vi "ConfigureDlg.vi"(8 "error in (no error)":errorcluster, 11 "SiemensDigitalEnergyMeter in":refnum<class "SiemensDigitalEnergyMeter.lvclass">) -> (0 "error out":errorcluster, 2 "Changed":bool, 3 "SiemensDigitalEnergyMeter out":refnum<class "SiemensDigitalEnergyMeter.lvclass">)   [LabVIEW 2018, in "SensorPlugins.lvlib" / "SiemensDigitalEnergyMeter.lvclass"]
doc: "This VI allows the user to configure the instrument using the provided panel and saves the instruments configuration to file, a new file, or cancels the entire operation."
uses:
  SiemensDigitalEnergyMeter.lvclass
  C:/Program Files (x86)/National Instruments/LabVIEW 2018/user.lib/NIST/BaseClasses/BasePlugin_class/BasePlugin.lvclass
  TypeDefinitions/SiemensDigitalEnergyMeterControls.ctl
  TypeDefinitions/MeasurementControls.ctl
  <userlib>/NIST/BaseClasses/BasePlugin_class/BasePlugin.lvclass/BasePlugin.ctl
  <userlib>/NIST/BaseClasses/BasePlugin_class/Accessors/Read PluginIniFilePath.vi
  <userlib>/NIST/BaseClasses/BasePlugin_class/Accessors/Write PluginIniFilePath.vi
  <vilib>/Utility/config.llb/NI_LVConfig.lvlib
panel:
  in  "MeasurementCluster":T1
  in  "Siemens Digital Energy Meter":T2 {"Measurement(s)" items=["kWh System"=4000, "kVARh System"=4007, "kVAh System"=4010, "kVA System"=4012, "Volts L1 to L2"=4018, "Volts L2 to L3"=4019, "Volts L1 to L2"=4020, "Line Frequency"=4021, "kW L1"=4028, "kW L2"=4029, "kW L3"=4030, "kVAR L1"=4037, "kVAR L2"=4038, "kVAR L3"=4039, "kVA L1"=4046, "kVA L2"=4047, "kVA L3"=4048, "Apparent PF L1"=4052, "Apparent PF L2"=4053, "Apparent PF L3"=4054, "Amps L1"=4055, "Amps L2"=4056, "Amps L3"=4057, "Volts L1 to Neutral"=4058, "Volts L2 to Neutral"=4059, "Volts L3 to Neutral"=4060, "Firmware Major Revision"=4068, "Firmware Minor Revision "=4069, "Model Number "=4200, "Serial Number"=4205, "Hardware ID"=4510]}
  in  "btnSaveAs":bool
  in  "btnSave":bool
  in  "btnCancel":bool
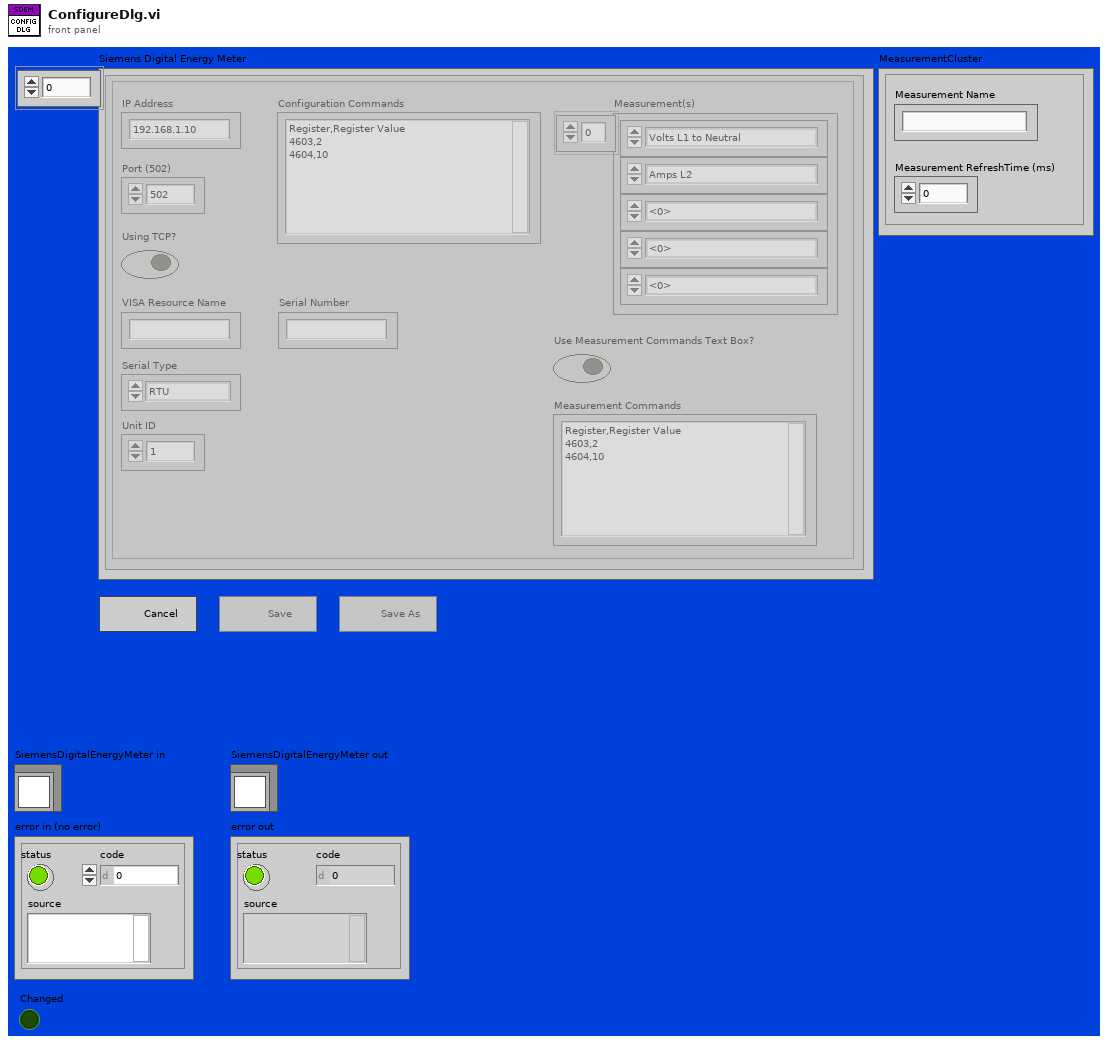
[diagram p1: front panel]
types:
  T1 = typedef "SensorPlugins.lvlib/SiemensDigitalEnergyMeter.lvclass/MeasurementControls.ctl" = cluster{"Measurement RefreshTime (ms)":u32, "Measurement Name":string}
  T2 = typedef "SensorPlugins.lvlib/SiemensDigitalEnergyMeter.lvclass/SiemensDigitalEnergyMeterControls.ctl" = cluster{"Measurement(s)":u16[], "Configuration Commands":string, "Use Measurement Commands Text Box?":bool, "Measurement Commands":string, "Connected?":bool, "Serial Number":string, "IP Address":string, "Port (502)":u16, "Unit ID":u8, "Serial Type":enum16{"RTU", "ASCII"}, "Using TCP?":bool, "VISA Resource Name":string}[]
  T3 = enum32{"Invalid", "Default", "Floating", "Floating/Auto-Hide", "Modal"}
  T4 = enum32{"Invalid", "Standard", "Closed", "Hidden", "Minimized", "Maximized"}
  T5 = enum8{"Enabled", "Disabled", "Disabled and Grayed Out"}
  T6 = cluster{"Measurement(s)":u16[], "Configuration Commands":string, "Use Measurement Commands Text Box?":bool, "Measurement Commands":string, "Connected?":bool, "Serial Number":string, "IP Address":string, "Port (502)":u16, "Unit ID":u8, "Serial Type":enum16{"RTU", "ASCII"}, "Using TCP?":bool, "VISA Resource Name":string}
  T7 = typedef "NI_LVConfig.lvlib/Config Data RefNum.ctl" = refnum<k1>
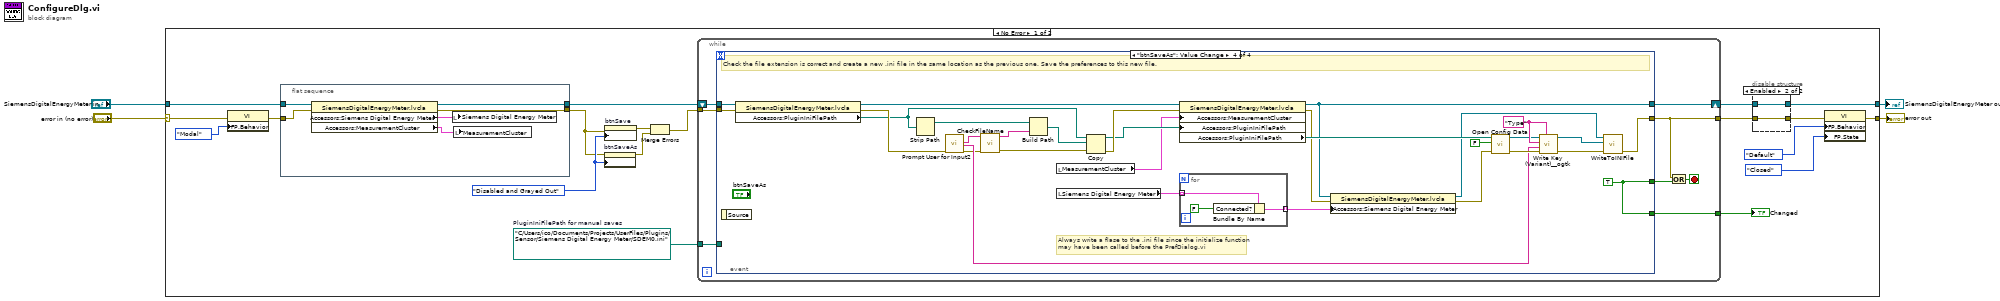
[diagram p0: block diagram]
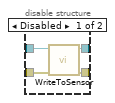
[diagram p2: hidden frame]
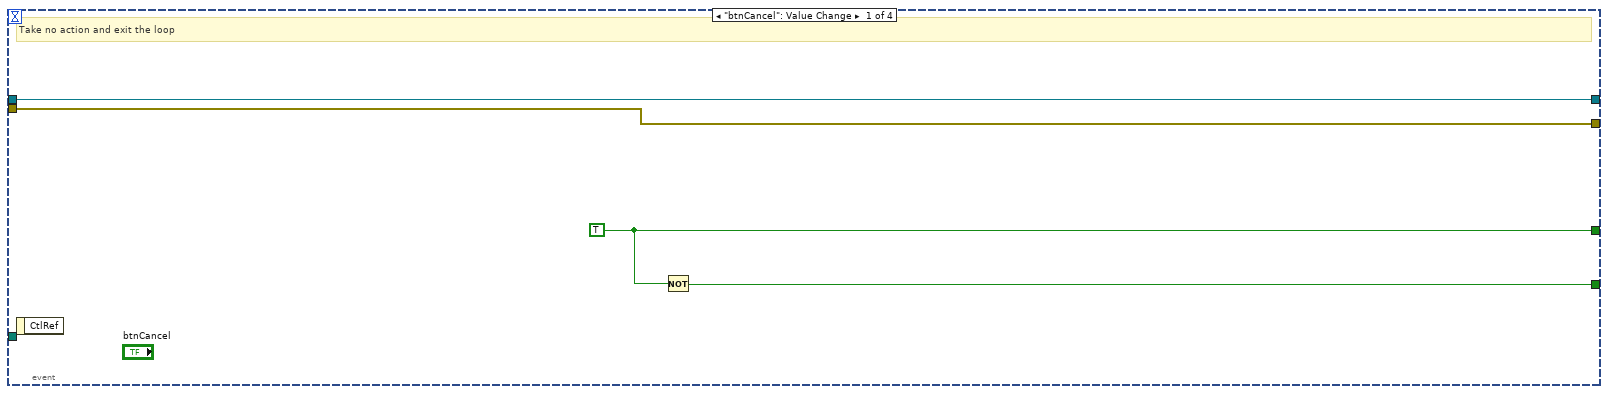
[diagram p3: hidden frame]
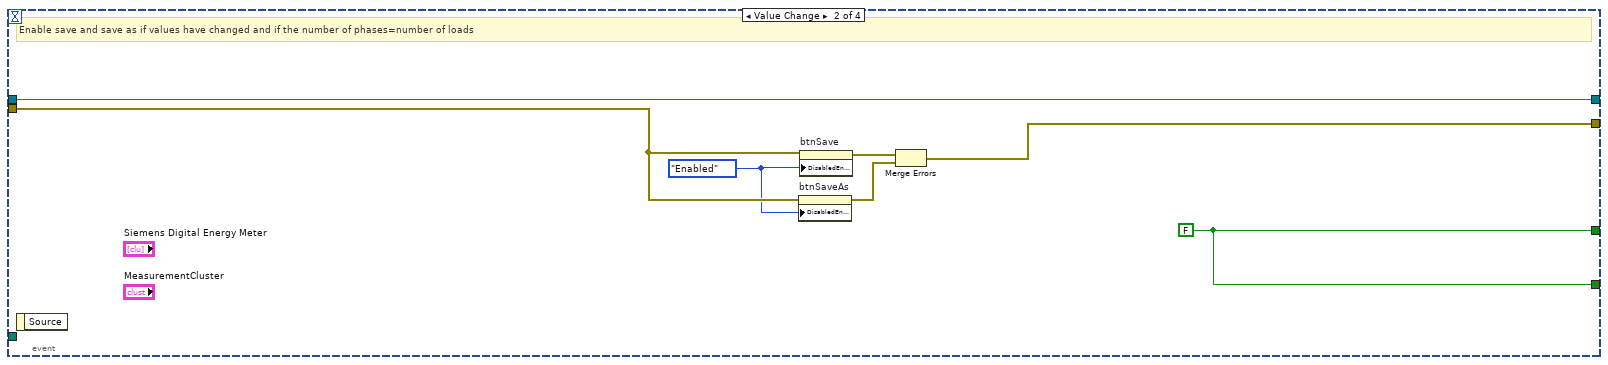
[diagram p4: hidden frame]
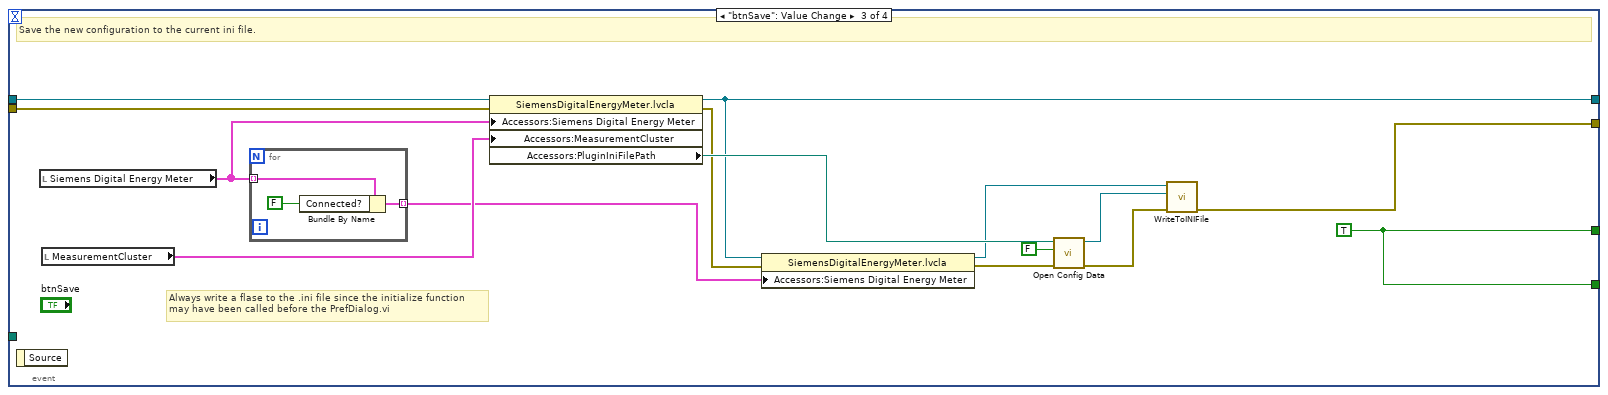
[diagram p5: hidden frame]
diagram:
  n1 = case shown="No Error" "error in (no error)" {
    selector: "error in (no error)" -> [w21 w106]
    tunnel: [w7 w107] -> w1
    tunnel: [w5 w106] -> w2
    tunnel: "SiemensDigitalEnergyMeter in" -> [w22 w107]
    frame No Error {
      w14 = T5."Disabled and Grayed Out" ("Disabled")
      w11 = path "C:/Users/ico/Documents/Projects/UserFiles/Plugins/Sensor/Siemens Digital Energy Meter/SDEM0.ini"  # PluginIniFilePath for manual saves
      n2 = property class="VI"(error in=w21, "FP.Behavior"=T3."Modal" ("Front Panel Window:Behavior")) -> (error out=w19:errorcluster)  [unwired: 1 in, 1 out]
      n3 = flat-sequence {
        tunnel: w22 -> [w34]
        tunnel: [w32] -> w18
        tunnel: [w31] -> w13
        tunnel: w19 -> [w35]
        frame #0 {
          n4 = property class="SiemensDigitalEnergyMeter.lvcla"(reference=w34, error in=w35) -> (reference out=w32:refnum<class "SiemensDigitalEnergyMeter.lvclass">, error out=w31:errorcluster, "Accessors:Siemens Digital Energy Meter"=w33:T2, "Accessors:MeasurementCluster"=w30:T1)
          n5 = local write "Siemens Digital Energy Meter"(w33) -> ()
          n6 = local write "MeasurementCluster"(w30) -> ()
        }
      }
      n7 = property on="btnSaveAs" class="Bool"(error in=w13, "DisabledEnum"=w14) -> (error out=w15:errorcluster)  [unwired: 1 in, 1 out]
      n8 = property on="btnSave" class="Bool"(error in=w13, "DisabledEnum"=w14) -> (error out=w16:errorcluster)  [unwired: 1 in, 1 out]
      n9 = Merge Errors(w16, w15) -> (w12:errorcluster)
      n10 = while {
        shift-right: [w42] -> w10
        shift-left: w18 -> [w43]
        tunnel: w12 -> [w41]
        tunnel: [w38] -> w9
        tunnel: [w40] -> w17
        tunnel: w11 -> [w36]
        stop <- w39 stop-if-true
        n11 = event shown="[3] \"btnSaveAs\": Value Change" {
          selector: _ -> [_ _ _ _]
          dyn-events: _ -> [_ _ _ _]
          timeout: _ -> [_ _ _ _]
          tunnel: w43 -> [w47 w51 w67 w88]
          tunnel: [w45 w54 w68 w101] -> w37
          tunnel: [w47 w51 w55 w74] -> w42
          tunnel: w41 -> [w46 w53 w64 w87]
          tunnel: [w46 w52 w65 w99] -> w38
          tunnel: [w44 w54 w68 w101] -> w40
          tunnel: w36 -> [_ _ _ _]
          event "btnCancel": Value Change {
            w45 = TRUE
            # "Take no action and exit the loop"
            n12 = event-data() -> ()  [unwired: 1 in, 1 out]
            n13 = Not(x=w45) -> (.not. x?=w44:bool)
          }
          event Value Change {
            w48 = T5."Enabled" ("Disabled")
            w54 = FALSE
            # "Enable save and save as if values have changed and if the number of phases=number of loads"
            n14 = event-data() -> ()  [unwired: 1 in, 1 out]
            n15 = property on="btnSaveAs" class="Bool"(error in=w53, "DisabledEnum"=w48) -> (error out=w50:errorcluster)  [unwired: 1 in, 1 out]
            n16 = property on="btnSave" class="Bool"(error in=w53, "DisabledEnum"=w48) -> (error out=w49:errorcluster)  [unwired: 1 in, 1 out]
            n17 = Merge Errors(w49, w50) -> (w52:errorcluster)
          }
          event "btnSave": Value Change {
            w68 = TRUE
            # "Always write a flase to the .ini file since the initialize function\nmay have been called before the PrefDialog.vi"
            # "Save the new configuration to the current ini file."
            n18 = event-data() -> ()  [unwired: 1 in, 1 out]
            n19 = local read "Siemens Digital Energy Meter"() -> (w61:T2)
            n20 = local read "MeasurementCluster"() -> (w62:T1)
            n21 = for {
              tunnel: w61 -> [w71] mode=indexing
              tunnel: [w72] -> w59 mode=indexing
              n22 = Bundle By Name(cluster=w71, "Connected?"=FALSE) -> (w72:T6)
            }
            n23 = property class="SiemensDigitalEnergyMeter.lvcla"(reference=w67, error in=w64, "Accessors:Siemens Digital Energy Meter"=w61, "Accessors:MeasurementCluster"=w62) -> (reference out=w55:refnum<class "SiemensDigitalEnergyMeter.lvclass">, error out=w60:errorcluster, "Accessors:PluginIniFilePath"=w63:path)
            n24 = property class="SiemensDigitalEnergyMeter.lvcla"(reference=w55, error in=w60, "Accessors:Siemens Digital Energy Meter"=w59) -> (reference out=w58:refnum<class "SiemensDigitalEnergyMeter.lvclass">, error out=w56:errorcluster)
            n25 = call <vilib>:"Open Config Data.vi"("error in (no error)"=w56, "create file if necessary (T)"=FALSE, "configuration file path"=w63) -> ("error out"=w57:errorcluster, "refnum"=w66:T7)  [unwired: 6 in, 1 out]
            n26 = call-dynamic "WriteToINIFile.vi"("error in (no error)"=w57, "Refnum in"=w66, "SiemensDigitalEnergyMeter in"=w58) -> ("error out"=w65:errorcluster)  [unwired: 7 in, 1 out]
          }
          event "btnSaveAs": Value Change {
            w98 = "Type" ("section (optional)")
            w101 = TRUE
            # "Always write a flase to the .ini file since the initialize function\nmay have been called before the PrefDialog.vi"
            # "Check the file extension is correct and create a new .ini file in the same location as the previous one. Save the preferences to this new file."
            n27 = event-data() -> ()  [unwired: 1 in, 1 out]
            n28 = property class="SiemensDigitalEnergyMeter.lvcla"(reference=w88, error in=w87) -> (reference out=w86:refnum<class "SiemensDigitalEnergyMeter.lvclass">, error out=w85:errorcluster, "Accessors:PluginIniFilePath"=w84:path)
            n29 = Strip Path(path=w84) -> (stripped path=w93:path)  [unwired: 1 out]
            n30 = call "Prompt User for Input2"("error in (no error)"=w85) -> ("File Name"=w80:string, "PluginType"=w83:string, "error out"=w79:errorcluster)  [unwired: 15 in, 1 out]
            n31 = call "CheckFileName.vi"("Error In"=w79, "File Name in"=w80) -> ("Error Out"=w81:errorcluster, "File Name out"=w82:string)  [unwired: 8 in]
            n32 = Build Path(base path=w93, name or relative path=w82) -> (appended path=w92:path)
            n33 = local read "MeasurementCluster"() -> (w78:T1)
            n34 = local read "Siemens Digital Energy Meter"() -> (w100:T2)
            n35 = Copy(8:w81, 10:w92, 11:w84) -> (0:w91:errorcluster, 3:w89:path)  [unwired: 2 in, 1 out]
            n36 = property class="SiemensDigitalEnergyMeter.lvcla"(reference=w86, error in=w91, "Accessors:MeasurementCluster"=w78, "Accessors:PluginIniFilePath"=w89) -> (reference out=w74:refnum<class "SiemensDigitalEnergyMeter.lvclass">, error out=w76:errorcluster, "Accessors:PluginIniFilePath"=w90:path)
            n37 = for {
              tunnel: w100 -> [w104] mode=indexing
              tunnel: [w105] -> w77 mode=indexing
              n38 = Bundle By Name(cluster=w104, "Connected?"=FALSE) -> (w105:T6)
            }
            n39 = property class="SiemensDigitalEnergyMeter.lvcla"(reference=w74, error in=w76, "Accessors:Siemens Digital Energy Meter"=w77) -> (reference out=w73:refnum<class "SiemensDigitalEnergyMeter.lvclass">, error out=w75:errorcluster)
            n40 = call <vilib>:"Open Config Data.vi"("error in (no error)"=w75, "create file if necessary (T)"=FALSE, "configuration file path"=w90) -> ("error out"=w96:errorcluster, "refnum"=w97:T7)  [unwired: 6 in, 1 out]
            n41 = call <userlib>:"Write Key (Variant)__ogtk.vi"("section"=w98, "error in (no error)"=w96, "key-value"=w83, "key (optional)"=w98, "refnum"=w97) -> ("error out"=w95:errorcluster, "refnum out"=w94:T7)  [unwired: 5 in]
            n42 = call-dynamic "WriteToINIFile.vi"("error in (no error)"=w95, "Refnum in"=w94, "SiemensDigitalEnergyMeter in"=w73) -> ("error out"=w99:errorcluster)  [unwired: 7 in, 1 out]
          }
        }
        n43 = Or(x=w38, y=w37) -> (x .or. y?=w39:bool)
      }
      "Changed" <- w17
      n44 = disable-structure shown="Enabled" {
        disable-tunnel: w10 -> [w27 w28]
        disable-tunnel: w9 -> [w26 w29]
        disable-tunnel: [w25 w29] -> w8
        disable-tunnel: [w24 w28] -> w7
        frame Disabled {
          n45 = call-dynamic "WriteToSensor.vi"("error in (no error)"=w26, "SiemensDigitalEnergyMeter in"=w27) -> ("error out"=w25:errorcluster, "SiemensDigitalEnergyMeter out"=w24:refnum<class "SiemensDigitalEnergyMeter.lvclass">)  [unwired: 8 in]
        }
        frame Enabled {
        }
      }
      n46 = property class="VI"(error in=w8, "FP.Behavior"=T3."Default" ("Front Panel Window:Behavior"), "FP.State"=T4."Closed" ("Front Panel Window:State")) -> (error out=w5:errorcluster)  [unwired: 1 in, 1 out]
    }
    frame Error {
    }
  }
  "error out" <- w2
  "SiemensDigitalEnergyMeter out" <- w1
